vi "Clear.vi"(8 "error in (no error)":errorcluster, 10 "Ctrl Sequences":string[](array[string]), 11 "front panel":refnum<vi>) -> (0 "error out":errorcluster, 3 "front panel out":refnum<vi>)   [LabVIEW 2018, in "NISAST VI Scripting.lvlib" / "VI.lvlib" / "Front Panel.lvlib"]
uses:
  Front Panel.lvlib
  Connector/Connector.lvlib
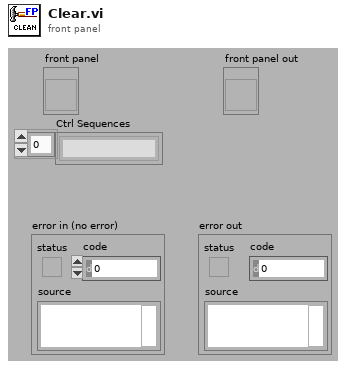
[diagram p1: front panel]
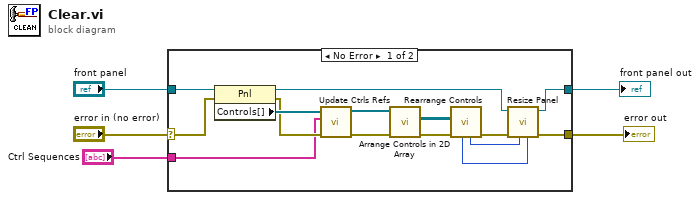
[diagram p0: block diagram]
diagram:
  n1 = case shown="No Error" "error in (no error)" {
    selector: "error in (no error)" -> [w17 w22]
    tunnel: [w15 w22] -> w4
    tunnel: "front panel" -> [w18 w21]
    tunnel: [w12 w21] -> w2
    tunnel: "Ctrl Sequences" -> [w6 _]
    frame No Error {
      n2 = property class="Pnl"(reference=w18, error in=w17) -> (reference out=w13:refnum<vi>, error out=w9:errorcluster, "Controls[]"=w10:refnum<vi>[])
      n3 = call "Update Ctrls Refs.vi"("error in"=w9, "Ctrl Sequences"=w6, "Controls[] in"=w10) -> ("error out"=w8:errorcluster, "Controls[] out"=w7:refnum<vi>[])  [unwired: 7 out]
      n4 = call "Arrange Controls in 2D Array.vi"("error in (no error)"=w8, "Controls[]"=w7) -> ("error out"=w20:errorcluster, "controls 2D[]"=w19:refnum<vi>[][])  [unwired: 1 in, 7 out]
      n5 = call "Rearrange Controls.vi"("error in"=w20, "controls references"=w19) -> ("error out"=w16:errorcluster, "panel width"=w14:i16, "panel height"=w11:i16)  [unwired: 1 in, 6 out]
      n6 = call "Resize Panel.vi"("panel height"=w11, "panel width"=w14, "error in"=w16, "Panel"=w13) -> ("error out"=w15:errorcluster, "Panel out"=w12:refnum<vi>)  [unwired: 2 in, 4 out]
    }
    frame Error {
    }
  }
  "error out" <- w4
  "front panel out" <- w2
